vi "InitPronyConfig.vi"(7 "Ring Refnum":refnum<vi>, 8 "error in (no error)":errorcluster, 10 "Prony Configuration":T1={"Lpmcon"=3, "Lpacon"=1, "Fbcon"=1, "LPOrd"={"Auto"=FALSE, "Val"=116}, "UTrimFreq"={"Auto"=FALSE, "Val"=20.0}, "LTrimFreq"={"Auto"=FALSE, "Val"=0.0}, "ResTrim"={"Auto"=FALSE, "Val"=1e-08}} {"Fbcon" items=["", "Forward", "Forward-Backward", "Backward"]; "Lpacon" items=["", "SVD with possible rank reduction", "QR reduction via LAPACK", "Total least squares via SVD"]; "Lpmcon" items=["", "Correlation", "Pre-windowed", "Covariance", "Post-windowed"]}, 11 "RingdownPlugin":refnum<class "RingdownPlugin.lvclass">=refnum) -> (0 "error out":errorcluster, 2 "Prony Configuration":T1 {"Fbcon" items=["", "Forward", "Forward-Backward", "Backward"]; "Lpacon" items=["", "SVD with possible rank reduction", "QR reduction via LAPACK", "Total least squares via SVD"]; "Lpmcon" items=["", "Correlation", "Pre-windowed", "Covariance", "Post-windowed"]}, 3 "RingdownPlugin":refnum<class "RingdownPlugin.lvclass">)   [LabVIEW 2014, in "AppPlugins.lvlib" / "RingdownPlugin.lvclass"]
uses:
  RingdownPlugin.lvclass
  PronyConfig.ctl
  PublicAPI/TypeDef/ePhase.ctl
  RingdownPlugin.lvclass/RingdownPlugin.ctl
  <vilib>/Utility/miscctls.llb/LVStringsAndValuesArrayTypeDef_U16.ctl
  Accessors/Read RingdownConfig.vi
  <vilib>/Utility/error.llb/Error Cluster From Error Code.vi
  <vilib>/ErrorRing/Error Ring.xnode
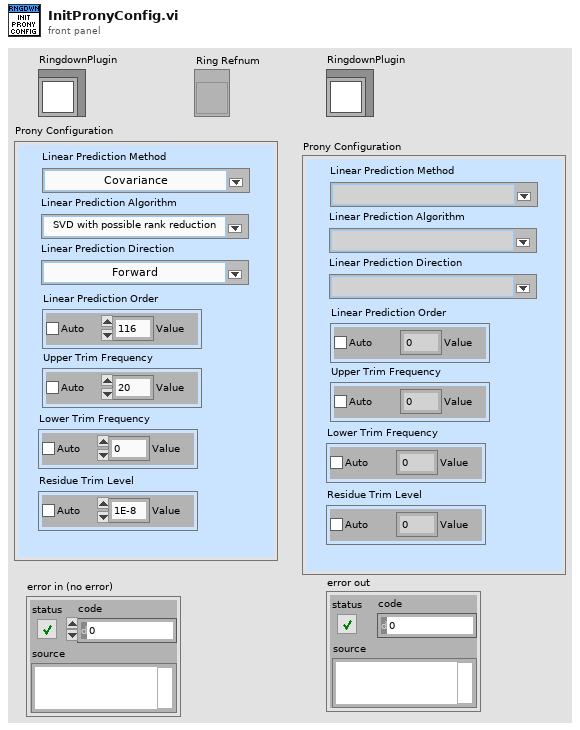
[diagram p1: front panel]
types:
  T1 = typedef "AppPlugins.lvlib/RingdownPlugin.lvclass/PronyConfig.ctl" = cluster{"Lpmcon":u16, "Lpacon":u16, "Fbcon":u16, "LPOrd":cluster{"Auto":bool, "Val":i32}, "UTrimFreq":cluster{"Auto":bool, "Val":dbl}, "LTrimFreq":cluster{"Auto":bool, "Val":dbl}, "ResTrim":cluster{"Auto":bool, "Val":dbl}}
  T2 = typedef "AppPlugins.lvlib/RingdownPlugin.lvclass/RingdownConfig.ctl" = cluster{"Config":cluster{"Addmod":i32, "Scalmod":i32, "Lpocon":i32, "Pircon":i32, "Dmodes":i32, "Lpmcon":u16, "Lpacon":u16, "Fbcon":u16, "Ordcon":i32, "Trimre":dbl, "Ftrimh":dbl, "Ftriml":dbl}, "Window":cluster{"StOffset":i32, "EndOffset":i32, "Length":i32}, "V index":i32, "I index":i32, "PosSeq":bool}
  T3 = cluster{"Addmod":i32, "Scalmod":i32, "Lpocon":i32, "Pircon":i32, "Dmodes":i32, "Lpmcon":u16, "Lpacon":u16, "Fbcon":u16, "Ordcon":i32, "Trimre":dbl, "Ftrimh":dbl, "Ftriml":dbl}
  T4 = typedef "AppPlugins.lvlib/RingdownPlugin.lvclass/ePhase.ctl" = u16
  T5 = typedef "LVStringsAndValuesArrayTypeDef_U16.ctl" = cluster{"String":string, "Value":u16}[]
  T6 = typedef "ePhase.ctl" = u16
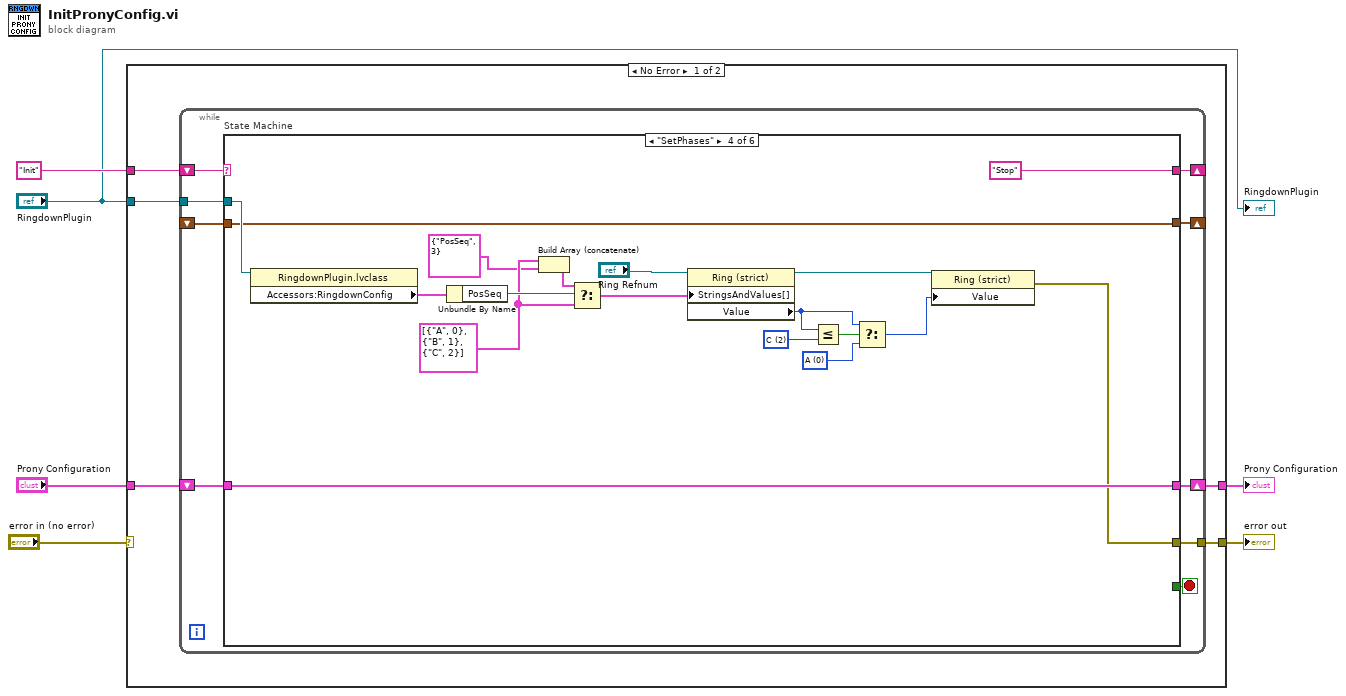
[diagram p0: block diagram]
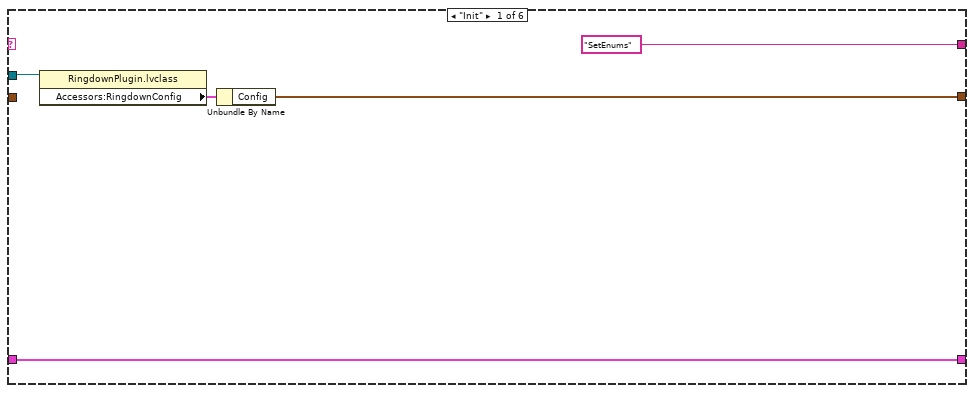
[diagram p2: hidden frame]
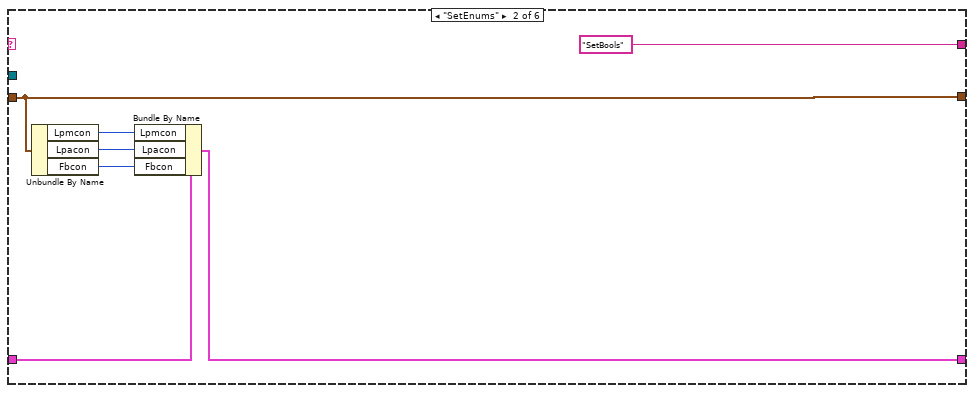
[diagram p3: hidden frame]
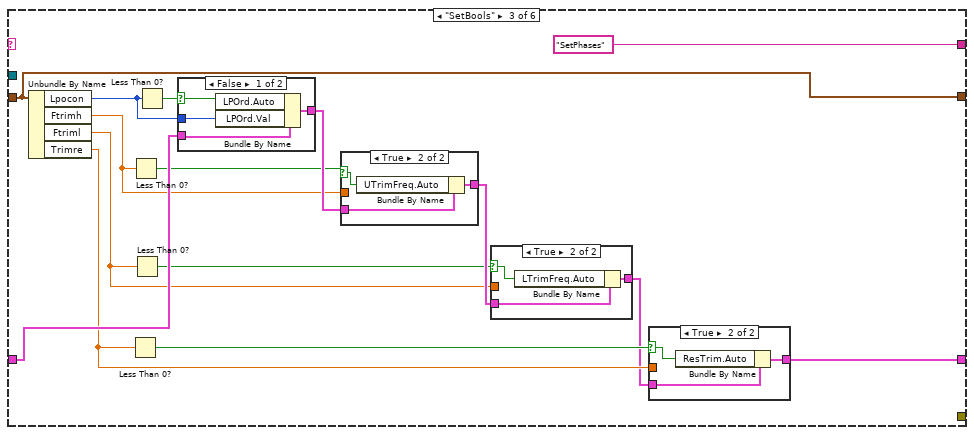
[diagram p4: hidden frame]
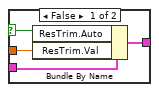
[diagram p5: hidden frame]
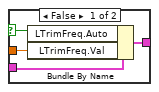
[diagram p6: hidden frame]
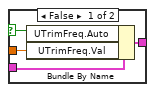
[diagram p7: hidden frame]
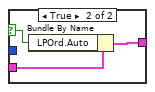
[diagram p8: hidden frame]
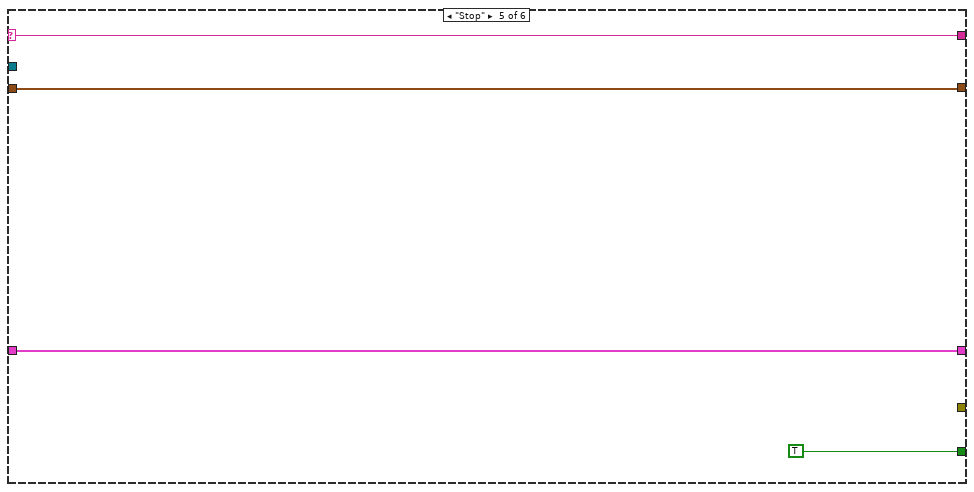
[diagram p9: hidden frame]
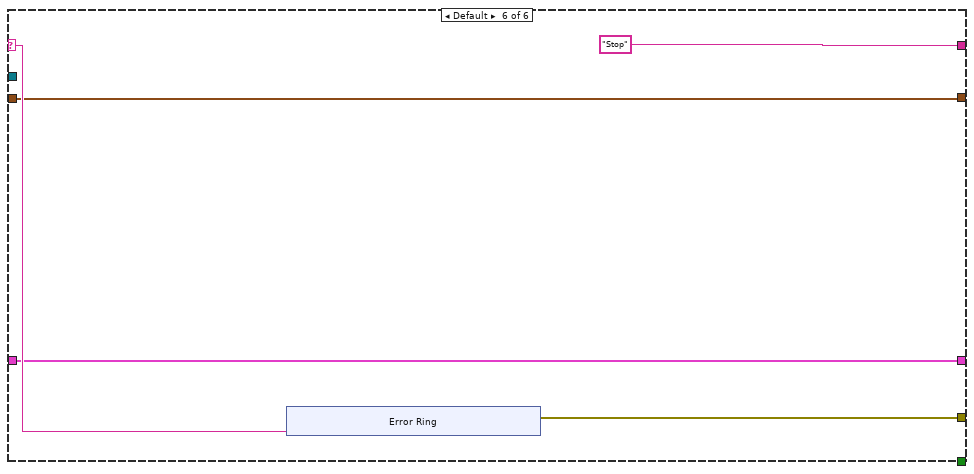
[diagram p10: hidden frame]
diagram:
  n1 = case shown="No Error" "error in (no error)" {
    selector: "error in (no error)" -> [_ w111]
    tunnel: "Init" -> [w11 _]
    tunnel: "Prony Configuration" -> [w10 w110]
    tunnel: "RingdownPlugin" -> [w9 _]
    tunnel: [w8 w110] -> w3
    tunnel: [w7 w111] -> w2
    frame No Error {
      n2 = while {
        shift-right: [w16] -> _
        shift-left: w11 -> [w20]
        shift-right: [w17] -> _
        shift-left: _ -> [w19]
        tunnel: w9 -> [w18]
        shift-right: [w14] -> w8
        shift-left: w10 -> [w15]
        tunnel: [w12] -> w7
        stop <- w13 stop-if-true
        n3 = case "State Machine" shown="\"SetPhases\"" w20 {
          selector: w20 -> [_ _ _ _ w96 w101]
          tunnel: w19 -> [_ w26 w33 w89 w95 w100]
          tunnel: w18 -> [w24 _ _ w93 _ _]
          tunnel: [w21 w26 w33 w89 w95 w100] -> w17
          tunnel: ["SetEnums" "SetBools" "SetPhases" "Stop" w96 "Stop"] -> w16
          tunnel: w15 -> [w22 w32 w45 w87 w94 w99]
          tunnel: [w22 w31 w34 w87 w94 w99] -> w14
          tunnel: [_ _ _ _ TRUE _] -> w13
          tunnel: [_ _ _ w80 _ w98] -> w12
          frame "Init" {
            n4 = property class="RingdownPlugin.lvclass"(reference=w24) -> ("Accessors:RingdownConfig"=w25:T2)  [unwired: 1 in, 2 out]
            n5 = Unbundle By Name(w25) -> ("Config"=w21:T3)
          }
          frame "SetEnums" {
            n6 = Unbundle By Name(w26) -> ("Lpmcon"=w30:u16, "Lpacon"=w29:u16, "Fbcon"=w28:u16)
            n7 = Bundle By Name(cluster=w32, "Lpmcon"=w30, "Lpacon"=w29, "Fbcon"=w28) -> (w31:T1)
          }
          frame "SetBools" {
            n8 = Unbundle By Name(w33) -> ("Lpocon"=w44:i32, "Ftrimh"=w42:dbl, "Ftriml"=w39:dbl, "Trimre"=w37:dbl)
            n9 = Less Than 0?(x=w37) -> (x < 0?=w36:bool)
            n10 = Less Than 0?(x=w42) -> (x < 0?=w41:bool)
            n11 = Less Than 0?(x=w39) -> (x < 0?=w38:bool)
            n12 = Less Than 0?(x=w44) -> (x < 0?=w46:bool)
            n13 = case shown="False" w46 {
              selector: w46 -> [w71 w75]
              tunnel: w45 -> [w72 w74]
              tunnel: [w69 w73] -> w43
              tunnel: w44 -> [w70 _]
              frame False {
                n14 = Bundle By Name(cluster=w72, "LPOrd.Auto"=w71, "LPOrd.Val"=w70) -> (w69:T1)
              }
              frame True {
                n15 = Bundle By Name(cluster=w74, "LPOrd.Auto"=w75) -> (w73:T1)
              }
            }
            n16 = case shown="True" w41 {
              selector: w41 -> [w64 w68]
              tunnel: w43 -> [w65 w67]
              tunnel: [w62 w66] -> w40
              tunnel: w42 -> [w63 _]
              frame False {
                n17 = Bundle By Name(cluster=w65, "UTrimFreq.Auto"=w64, "UTrimFreq.Val"=w63) -> (w62:T1)
              }
              frame True {
                n18 = Bundle By Name(cluster=w67, "UTrimFreq.Auto"=w68) -> (w66:T1)
              }
            }
            n19 = case shown="True" w38 {
              selector: w38 -> [w57 w61]
              tunnel: w40 -> [w58 w60]
              tunnel: [w55 w59] -> w35
              tunnel: w39 -> [w56 _]
              frame False {
                n20 = Bundle By Name(cluster=w58, "LTrimFreq.Auto"=w57, "LTrimFreq.Val"=w56) -> (w55:T1)
              }
              frame True {
                n21 = Bundle By Name(cluster=w60, "LTrimFreq.Auto"=w61) -> (w59:T1)
              }
            }
            n22 = case shown="True" w36 {
              selector: w36 -> [w50 w54]
              tunnel: w35 -> [w51 w53]
              tunnel: [w48 w52] -> w34
              tunnel: w37 -> [w49 _]
              frame False {
                n23 = Bundle By Name(cluster=w51, "ResTrim.Auto"=w50, "ResTrim.Val"=w49) -> (w48:T1)
              }
              frame True {
                n24 = Bundle By Name(cluster=w53, "ResTrim.Auto"=w54) -> (w52:T1)
              }
            }
          }
          frame "SetPhases" {
            w76 = T4 0 items=["A", "B", "C", "PosSeq"] ("y")
            w82 = T4 2 items=["A", "B", "C", "PosSeq"] ("y")
            w86 = T5 [{"String"="A", "Value"=0}, {"String"="B", "Value"=1}, {"String"="C", "Value"=2}] ("Strings And Values []")
            n25 = property class="RingdownPlugin.lvclass"(reference=w93) -> ("Accessors:RingdownConfig"=w92:T2)  [unwired: 1 in, 2 out]
            n26 = Unbundle By Name(w92) -> ("PosSeq"=w91:bool)
            n27 = Build Array (concatenate)(w86, cluster{"String":string, "Value":i32} {"String"="PosSeq", "Value"=3}) -> (w90:cluster{"String":string, "Value":i32}[])
            n28 = Select(t=w90, s=w91, f=w86) -> (s? t:f=w84:cluster{"String":string, "Value":i32}[])
            n29 = property class="Ring (strict)"(reference="Ring Refnum", "StringsAndValues[]"=w84) -> (reference out=w81:refnum<vi>, "Value"=w78:T6)  [unwired: 1 in, 1 out]
            n30 = Less Or Equal?(x=w78, y=w82) -> (x <= y?=w77:bool)
            n31 = Select(t=w78, s=w77, f=w76) -> (s? t:f=w79:T4)
            n32 = property class="Ring (strict)"(reference=w81, "Value"=w79) -> (error out=w80:errorcluster)  [unwired: 1 in, 1 out]
          }
          frame "Stop" {
          }
          frame Default {
            n33 = xnode "Error Ring"("parameter 0"=w101) -> ("error out"=w98:errorcluster)
          }
        }
      }
    }
    frame Error {
    }
  }
  "Prony Configuration" <- w3
  "error out" <- w2
  "RingdownPlugin" <- "RingdownPlugin"
